vi "Count.vi"(8 "error in (no error)":errorcluster, 11 "Store in":refnum<class "Store.lvclass">) -> (0 "error out":errorcluster, 2 "Size":i32, 3 "Store out":refnum<class "Store.lvclass">)   [LabVIEW 2018, in "Application.lvlib" / "Store.lvclass"]
uses:
  Store.lvclass
  Store.lvclass/Store.ctl
  Dictionary Class/Dictionary.lvclass/Dictionary.ctl
  Dictionary Class/VIs/Get Data DVR.vi
  Dictionary Class/Dictionary.lvclass
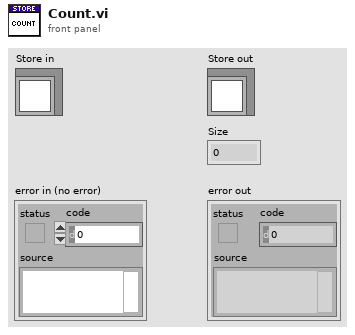
[diagram p1: front panel]
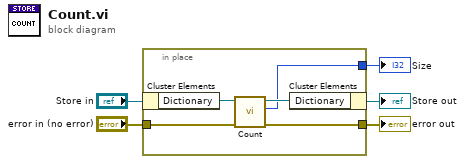
[diagram p0: block diagram]
diagram:
  n1 = in-place {
    in-place-border: [w8] -> w1
    in-place-border: "error in (no error)" -> [w7]
    in-place-border: [w6] -> w2
    n2 = in-place-cluster #1("Store in") -> ("Dictionary"=w10:refnum<class "Dictionary.lvclass">)
    n3 = call "Count.vi"("error in (no error)"=w7, "Dictionary in"=w10) -> ("error out"=w6:errorcluster, "Size"=w8:i32, "Dictionary out"=w9:refnum<class "Dictionary.lvclass">)  [unwired: 7 in]
    n4 = in-place-cluster #1("Dictionary"=w9) -> (→"Store out":refnum<class "Store.lvclass">)
  }
  "error out" <- w2
  "Size" <- w1
